vi "CMRR.vi"(11 "数组":dbl[](array[numeric])) -> (3 "KCMRR":dbl=118.45179628787717)   [LabVIEW 2019]
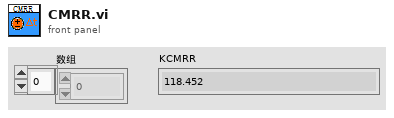
[diagram p1: front panel]
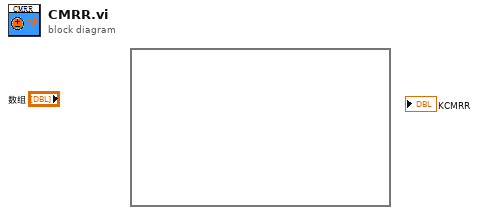
[diagram p0: block diagram]
diagram:
  n1 = formula code=""() -> ()
